vi "Renew Search Results.vi"(8 "error in (no error)":errorcluster, 10 "QDFunctionsData":variant[][](array[variant]), 11 "ScriptDialog in":refnum<class "ScriptDialog.lvclass">) -> (0 "error out":errorcluster, 3 "ScriptDialog out":refnum<class "ScriptDialog.lvclass">)   [LabVIEW 2015, in "ScriptDialog.lvclass"]
uses:
  ScriptDialog.lvclass
  QDFunctions/Implements/NormalQDFunc/NormalQDFunc.lvclass
  ScriptDialog.lvclass/ScriptDialog.ctl
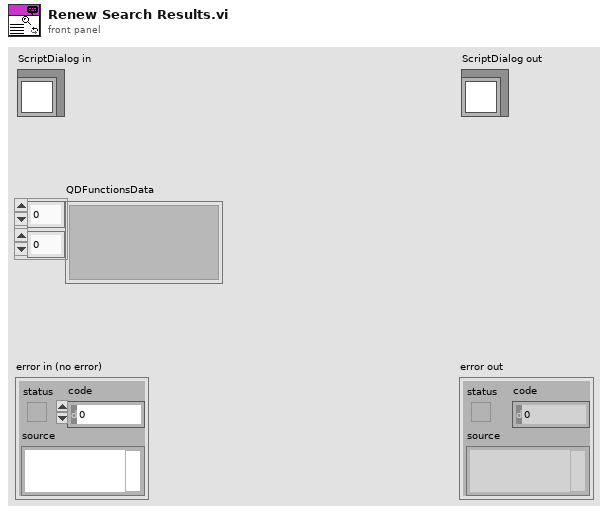
[diagram p1: front panel]
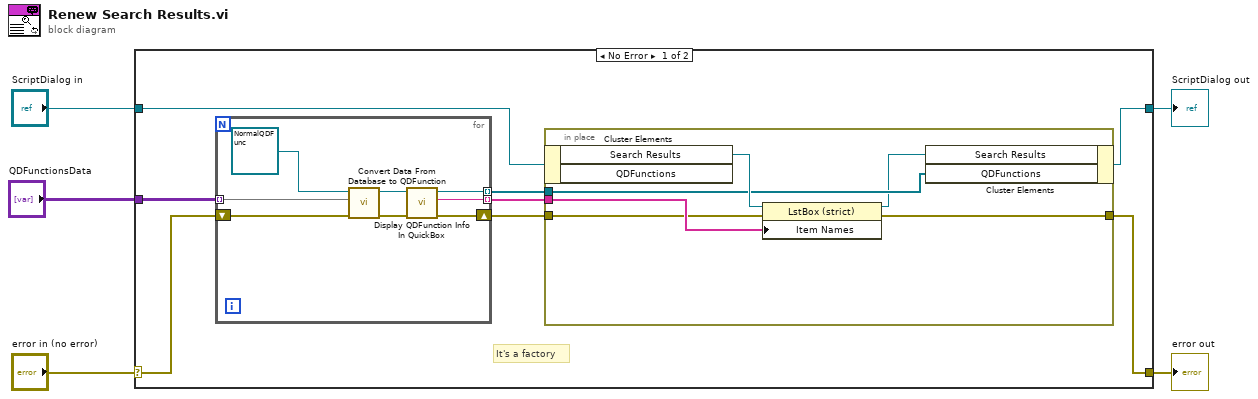
[diagram p0: block diagram]
diagram:
  n1 = case shown="No Error" "error in (no error)" {
    selector: "error in (no error)" -> [w7 w29]
    tunnel: [w6 w29] -> w4
    tunnel: [w8 w28] -> w2
    tunnel: "ScriptDialog in" -> [w12 w28]
    tunnel: "QDFunctionsData" -> [w13 _]
    frame No Error {
      # "It's a factory"
      n2 = for {
        tunnel: w13 -> [w27] mode=indexing
        tunnel: [w23] -> w9 mode=indexing
        tunnel: [w21] -> w11 mode=indexing
        shift-right: [w22] -> w10
        shift-left: w7 -> [w26]
        n3 = call-dynamic "Convert Data From Database to QDFunction.vi"("error in (no error)"=w26, "FetchedData"=w27, "NormalQDFunc in"=refnum<class "NormalQDFunc.lvclass"> refnum ("NormalQDFunc")) -> ("error out"=w24:errorcluster, "NormalQDFunc out"=w25:refnum<class "NormalQDFunc.lvclass">)  [unwired: 7 in]
        n4 = call-dynamic "Display QDFunction Info In QuickBox.vi"("error in (no error)"=w24, "NormalQDFunc in"=w25) -> ("error out"=w22:errorcluster, "Content For Display"=w21:string, "NormalQDFunc out"=w23:refnum<class "NormalQDFunc.lvclass">)  [unwired: 7 in]
      }
      n5 = in-place {
        in-place-border: w11 -> [w18]
        in-place-border: w10 -> [w17]
        in-place-border: w9 -> [w16]
        in-place-border: [w14] -> w6
        n6 = in-place-cluster #1(w12) -> ("Search Results"=w19:refnum<vi>)  [unwired: 1 out]
        n7 = property class="LstBox (strict)"(reference=w19, error in=w17, "Item Names"=w18) -> (reference out=w15:refnum<vi>, error out=w14:errorcluster)
        n8 = in-place-cluster #1("Search Results"=w15, "QDFunctions"=w16) -> (w8:refnum<class "ScriptDialog.lvclass">)
      }
    }
    frame Error {
    }
  }
  "error out" <- w4
  "ScriptDialog out" <- w2
